vi "testPy.vi"() -> ()   [LabVIEW 2019]
panel:
  out "Tf":dbl
  in  "Tc":dbl
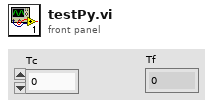
[diagram p1: front panel]
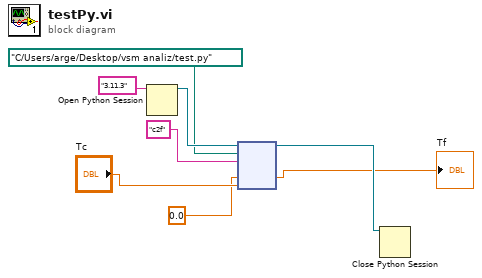
[diagram p0: block diagram]
diagram:
  n1 = Open Python Session(python version="3.11.3" ("Python version")) -> (session out=w7:refnum<k35>)  [unwired: 2 in, 1 out]
  n2 = node(w7, path "C:/Users/arge/Desktop/vsm analiz/test.py" ("module path"), "c2f" ("function name"), 0.0, "Tc") -> (w3:refnum<k35>, →"Tf":dbl)  [unwired: 2 in, 3 out]
  n3 = Close Python Session(session in=w3) -> ()  [unwired: 1 in, 1 out]
